vi "例4.15局部变量读取循环结构外的数据.vi"() -> ()   [LabVIEW 2017]
panel:
  in  "停止":bool
  out "Y":dbl
  in  "X":dbl
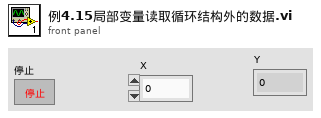
[diagram p1: front panel]
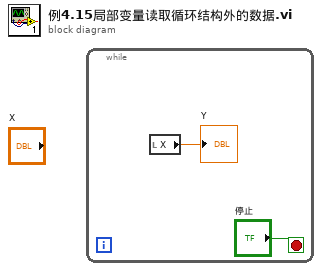
[diagram p0: block diagram]
diagram:
  n1 = while {
    stop <- "停止" stop-if-true
    n2 = local read "X"() -> (→"Y":dbl)
  }
